vi "Do.vi"(8 "error in (no error)":errorcluster, 10 "Actor in":refnum<class "Actor.lvclass">, 11 "Result Data Update the Self Msg":refnum<class "Result Data Update the Self Msg.lvclass">) -> (0 "error out":errorcluster, 2 "Actor out":refnum<class "Actor.lvclass">)   [LabVIEW 2023, in "Data Analysis.lvlib" / "Error Log.lvlib" / "Result Data Update the Self Msg.lvclass"]
doc: "This VI delivers the message to the actor by calling the appropriate method(s) on the actor."
uses:
  Result Data Update the Self Msg.lvclass
  Result Data Update the Self Msg.lvclass/Result Data Update the Self Msg.ctl
  5815967d-5168-4d26-9918-2f4b9d8eefc9.vi
  Error Log/Error Log.lvclass
  <vilib>/ActorFramework/Actor/Actor.lvclass
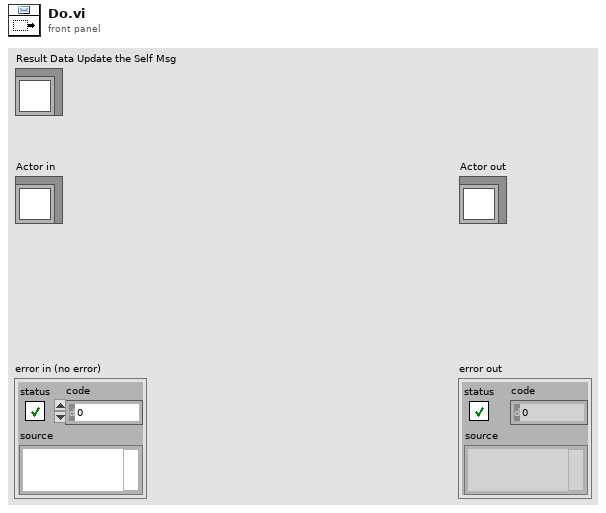
[diagram p1: front panel]
types:
  T1 = typedef "Data Analysis.lvlib/Report.ctl" = cluster{"Schema":string, "Test Socket":string, "Start Test Cycle":string, "Stop Test Cycle":string, "Test Mode":string, "Frame Type":string}
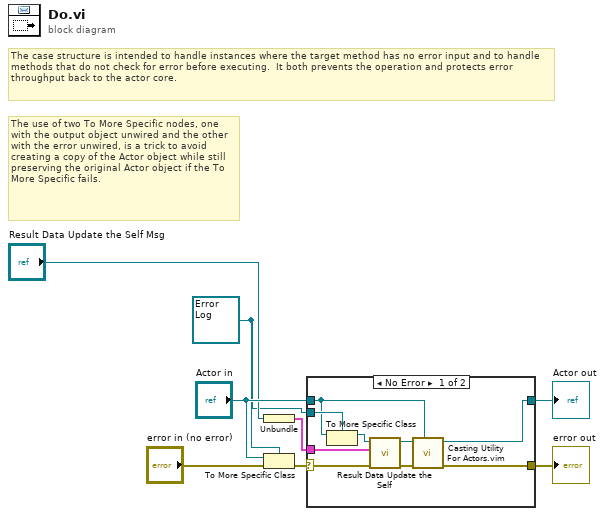
[diagram p0: block diagram]
diagram:
  w3 = refnum<class "Error Log.lvclass"> refnum ("Actor in")
  # "The use of two To More Specific nodes, one with the output object unwired and the other with the error unwired, is a trick to avoid creating a copy of the Actor object while still preserving the original Actor object if the To More Specific fails."
  # "The case structure is intended to handle instances where the target method has no error input and to handle methods that do not check for error before executing.  It both prevents the operation and protects error throughput back to the actor core."
  n1 = Unbundle("Result Data Update the Self Msg") -> (w1:T1)
  n2 = To More Specific Class(target class=w3, reference="Actor in", error in="error in (no error)") -> (error out=w2:errorcluster)  [unwired: 1 out]
  n3 = case shown="No Error" w2 {
    selector: w2 -> [w17 w19]
    tunnel: [w11 w19] -> w8
    tunnel: [w12 w18] -> w7
    tunnel: "Actor in" -> [w14 w18]
    tunnel: w3 -> [w15 _]
    tunnel: w1 -> [w9 _]
    frame No Error {
      n4 = To More Specific Class(target class=w15, reference=w14) -> (specific class reference=w16:refnum<class "Error Log.lvclass">)  [unwired: 1 in, 1 out]
      n5 = call "Result Data Update the Self.vi"("error in (no error)"=w17, "Report Data"=w9, "Error Log in"=w16) -> ("error out"=w10:errorcluster, "Error Log out"=w13:refnum<class "Error Log.lvclass">)  [unwired: 7 in]
      n6 = call "Casting Utility For Actors.vim"("type"=w14, "error in (no error)"=w10, "Actor in"=w13) -> ("error out"=w11:errorcluster, "Actor out"=w12:refnum<class "Actor.lvclass">)  [unwired: 7 in]
    }
    frame Error {
      # "If type check fails, pass the original object out again."
    }
  }
  "error out" <- w8
  "Actor out" <- w7
